vi "ReadHeater.vi"(3 "error in (no error)":errorcluster, 5 "VISA resource name":refnum<visa-resource-name>="COM19") -> (0 "error out":errorcluster, 1 "Power":string="t:   19.57 C\r\n", 2 "VISA resource name":refnum<visa-resource-name>="COM3")   [LabVIEW 2017]
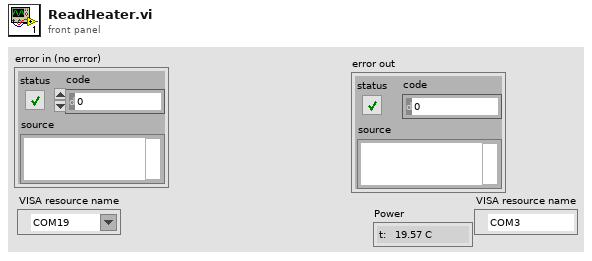
[diagram p1: front panel]
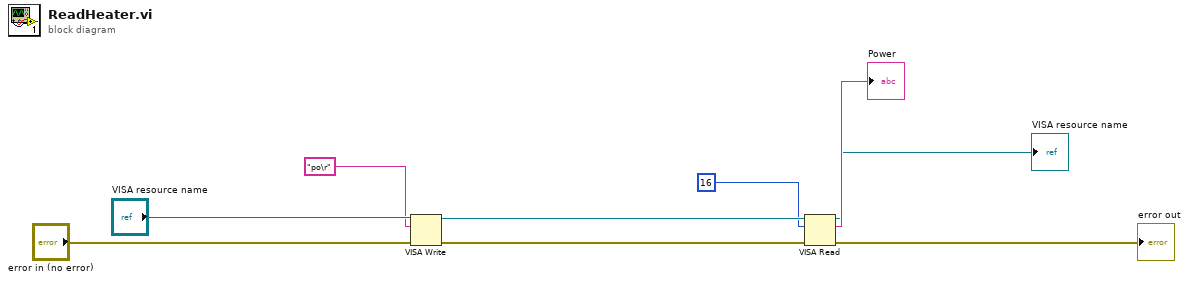
[diagram p0: block diagram]
diagram:
  n1 = VISA Write(VISA resource name="VISA resource name", write buffer="po\r", error in (no error)="error in (no error)") -> (VISA resource name out=w7:refnum<visa-resource-name>, error out=w6:errorcluster)  [unwired: 1 out]
  n2 = VISA Read(VISA resource name=w7, byte count=16, error in (no error)=w6) -> (VISA resource name out=→"VISA resource name":refnum<visa-resource-name>, read buffer=→"Power":string, error out=→"error out":errorcluster)  [unwired: 1 out]
